vi "General Error Handler - show previous state.vi"(8 "error in (no error)":errorcluster, 10 "Previous State":string, 11 "Loop Select":enum16{"Event Loop -", "Async Loop -"}(ring)) -> (0 "error out":errorcluster, 2 "resulting string":string)   [LabVIEW 2019]
uses:
  <vilib>/Utility/error.llb/DialogType.ctl
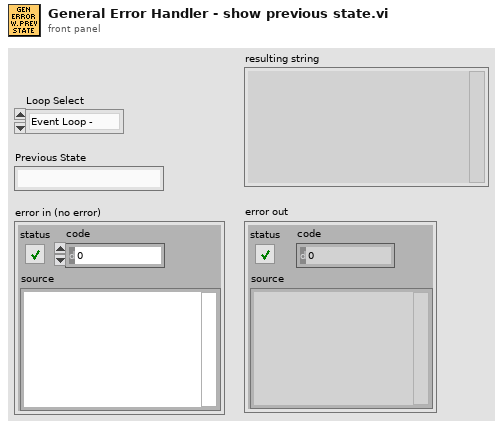
[diagram p1: front panel]
types:
  T1 = typedef "DialogType.ctl" = u16
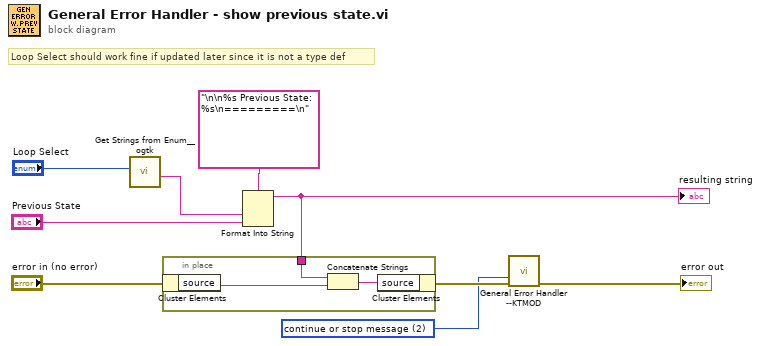
[diagram p0: block diagram]
diagram:
  w1 = T1 2 items=["no dialog", "OK message", "continue or stop message", "OK message + warnings", "continue/stop + warnings"] ("type of dialog (OK msg:1)")
  # "Loop Select should work fine if updated later since it is not a type def"
  n1 = call <userlib>:"Get Strings from Enum__ogtk.vi"("Enum"="Loop Select") -> ("String Value"=w6:string)  [unwired: 7 in, 3 out]
  n2 = Format Into String(format string="\n\n%s Previous State: %s\n=========\n", w6, "Previous State") -> (resulting string=w2:string)  [unwired: 2 in, 1 out]
  "resulting string" <- w2
  n3 = in-place {
    in-place-border: w2 -> [w11]
    n4 = in-place-cluster #1("error in (no error)") -> ("source"=w12:string)
    n5 = Concatenate Strings(w11, w12) -> (w10:string)
    n6 = in-place-cluster #1("source"=w10) -> (w3:errorcluster)
  }
  n7 = call "General Error Handler --KTMOD.vi"("type of dialog (OK msg:1)"=w1, "error in (no error)"=w3) -> ("error out"=→"error out":errorcluster)  [unwired: 9 in, 4 out]
